vi "retrieveNewData.vi"(8 "error in (no error)":errorcluster, 10 "model":refnum<class "Model.lvclass">, 11 "DisabledState in":refnum<class "DisabledState.lvclass">) -> (0 "error out":errorcluster, 2 "model 2":refnum<class "Model.lvclass">, 3 "DisabledState out":refnum<class "DisabledState.lvclass">)   [LabVIEW 2015, in "DisabledState.lvclass"]
uses:
  DisabledState.lvclass
  Model/Model/Model.lvclass
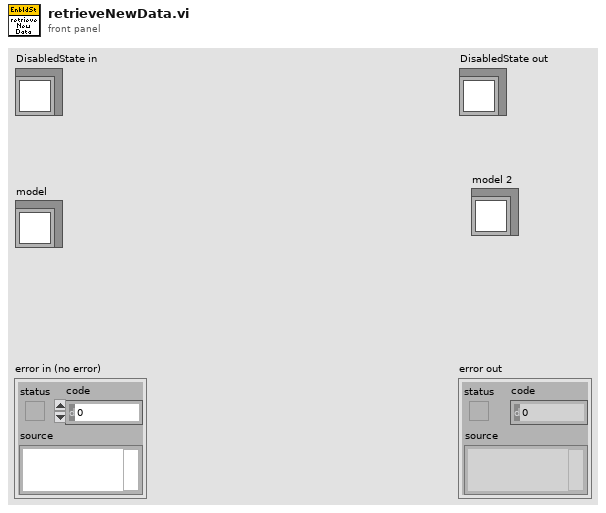
[diagram p1: front panel]
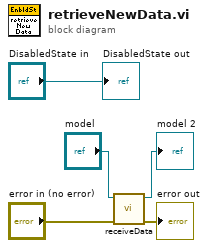
[diagram p0: block diagram]
diagram:
  n1 = call "receiveData.vi"("error in (no error)"="error in (no error)", "Model in"="model") -> ("error out"=→"error out":errorcluster, "Model out"=→"model 2":refnum<class "Model.lvclass">)  [unwired: 8 in]
  "DisabledState out" <- "DisabledState in"
